vi "Z Domain to Spectral Domain Bandwidth.vi"(9 "Samples":dbl format="%#_13g", 10 "Window Width":dbl format="%#_13g", 11 "Depth":dbl format="%#_13g") -> (2 "Low Pass Freq (scaled)":dbl, 3 "High Pass Freq (Scaled)":dbl)   [LabVIEW 2014]
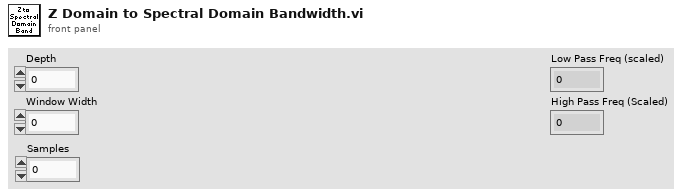
[diagram p1: front panel]
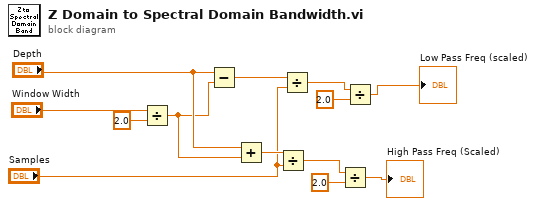
[diagram p0: block diagram]
diagram:
  n1 = Divide(x="Window Width", y=2.0) -> (x/y=w10:dbl)
  n2 = Subtract(x="Depth", y=w10) -> (x-y=w9:dbl)
  n3 = Add(x="Depth", y=w10) -> (x+y=w8:dbl)
  n4 = Divide(x=w8, y="Samples") -> (x/y=w5:dbl)
  n5 = Divide(x=w9, y="Samples") -> (x/y=w2:dbl)
  n6 = Divide(x=w5, y=2.0) -> (x/y=→"High Pass Freq (Scaled)":dbl)
  n7 = Divide(x=w2, y=2.0) -> (x/y=→"Low Pass Freq (scaled)":dbl)
